vi "main.vi"() -> ()   [LabVIEW 2013]
uses:
  measurement/measurement sweep parameter.ctl
  devices/magnet/magnet polar field.ctl
  devices/magnet/AMI reading polar field.ctl
  app/app global state actions.ctl
  <vilib>/Utility/error.llb/DialogType.ctl
  config.vi
panel:
  in  "Ramp to zero and switch off \nswitch heaters after measurement?":bool=TRUE
  out "Actual T (K)":dbl format="%#_4g"
  out "Current Magnetic\nField\n(430 TCP reading)":T1 {"phi (deg)" format="%#_4g"; "magnitude (T)" format="%#_4g"}
  in  "error in (no error)":errorcluster
  out "Log":string
  out "Current Magnetic Field\n(Gaussmeter reading)":T2 {"theta" format="%#_3g"; "phi" format="%#_3g"; "magnitude" format="%#_3g"}
  out "VNA Sweeping":bool
  out "Magnet Ramping":bool
  out "Sweep Increment":string
  out "Sweep Range":string
  out "Sweep Parameter":T3
  out "Current sweep":string
  in  "Measurement Folder (no backslash at the end)":path=path "D:/UserData/istasinopoulos/VTI/Cu2OSeO3/VTG_1_11_2_14072016/measurement2"
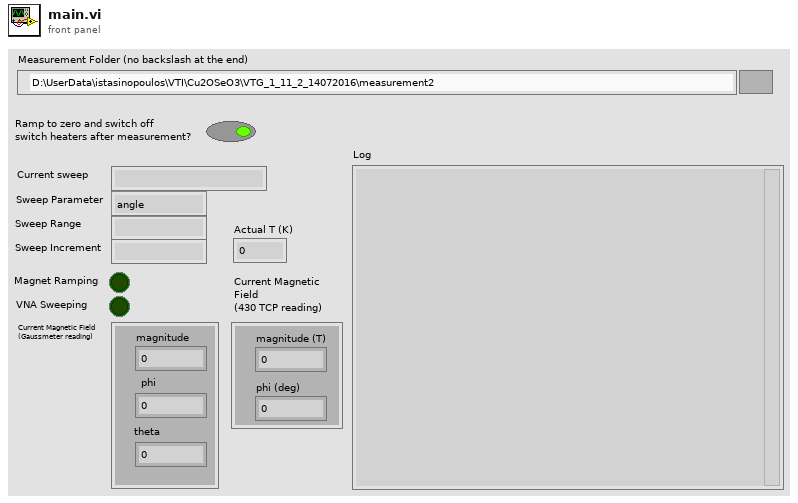
[diagram p1: front panel]
types:
  T1 = typedef "AMI reading polar field.ctl" = cluster{"magnitude (T)":dbl, "phi (deg)":dbl}
  T2 = typedef "magnet polar field.ctl" = cluster{"magnitude":dbl, "phi":dbl, "theta":dbl}
  T3 = typedef "measurement sweep parameter.ctl" = enum16{"angle", "magnetic field"}
  T4 = cluster{"freq start (Hz)":dbl, "freq stop (Hz)":dbl, "power (dBm)":i32, "IF bandwidth (Hz)":dbl, "no. points":i32, "calibration name":string, "SX1":bool, "SX2":bool}
  T5 = typedef "app global state actions.ctl" = enum16{"set field reached", "get cluster", "set cluster", "set current sweep", "set field value", "set 430 TCP reading", "set ramping", "set sweeping", "append log", "clear log", "set finished"}
  T6 = typedef "app global state control.ctl" = cluster{"current field value":T2, "field ramping":bool, "vna sweeping":bool, "Log Messages":string, "current sweep":T7, "measurement finished":bool, "Current Magnetic Field\n(430 TCP reading)":cluster{"magnitude (T)":dbl, "phi (deg)":dbl}, "field was reached":bool}
  T7 = typedef "measconfig cluster.ctl" = cluster{"sweep parameter":T3, "sweep start":dbl, "sweep stop":dbl, "sweep increment":dbl, "temperature":dbl, "path":path, "magnet initial":T2, "magnet reference":T2, "const phi?":bool, "delta phi (deg)":dbl, "delta H (mT)":dbl, "const phi init field?":bool}
  T8 = typedef "DialogType.ctl" = u16
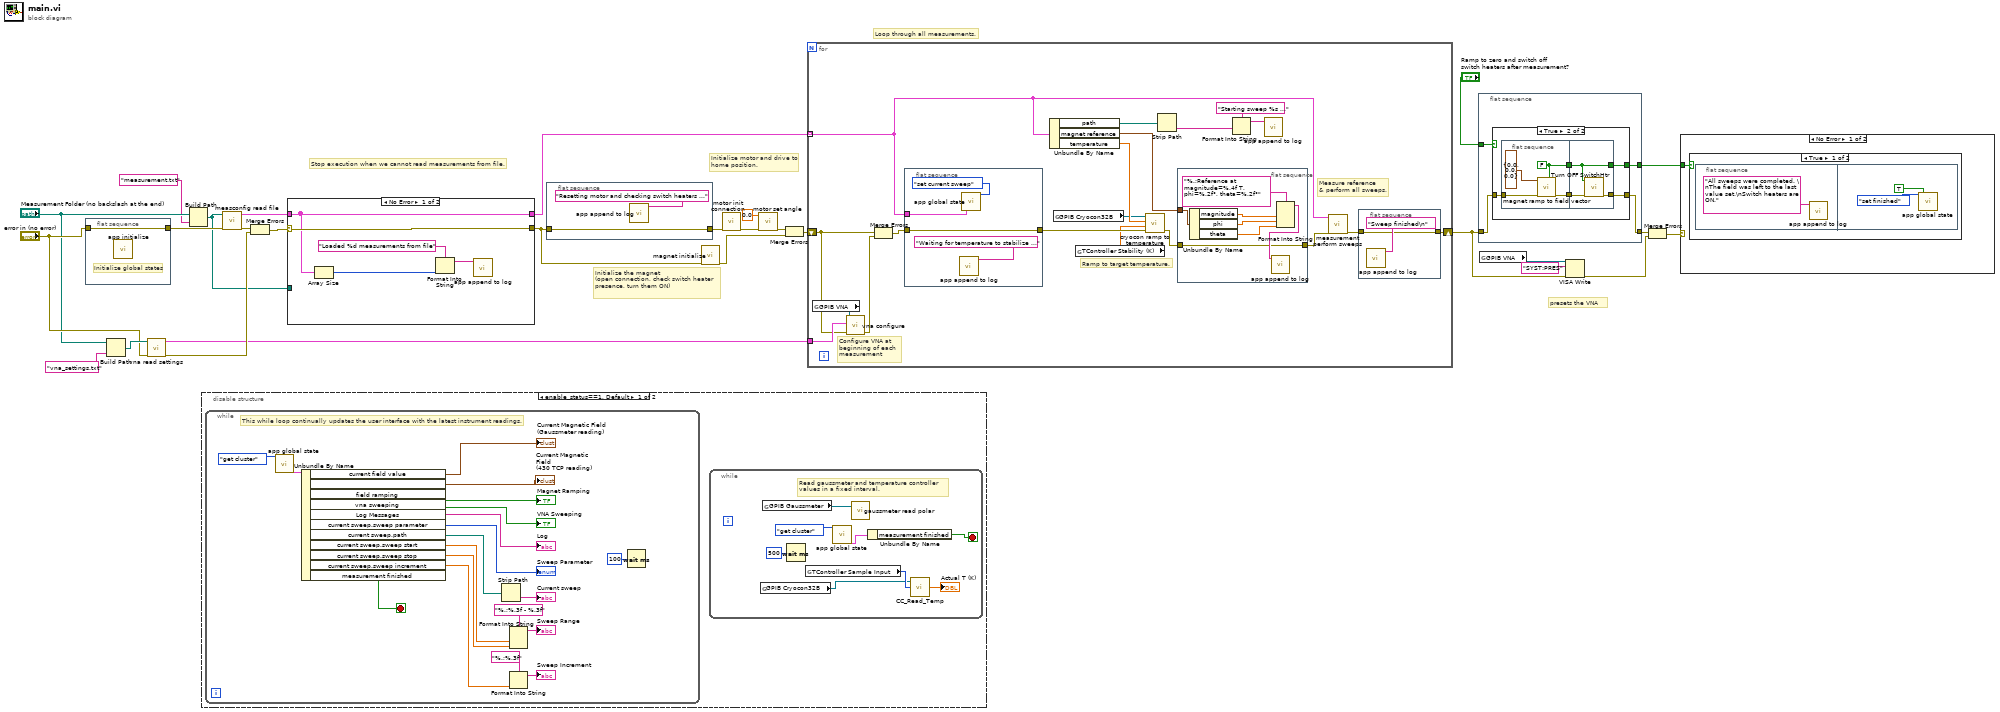
[diagram p0: block diagram]
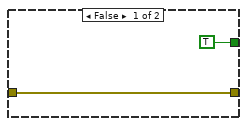
[diagram p2: hidden frame]
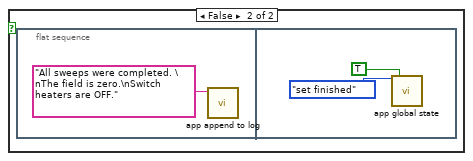
[diagram p4: hidden frame]
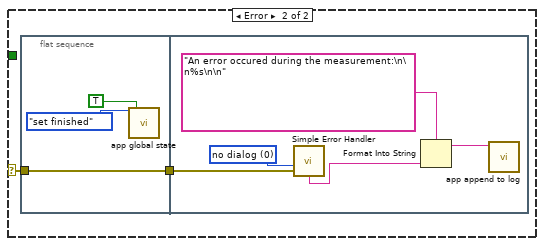
[diagram p5: hidden frame]
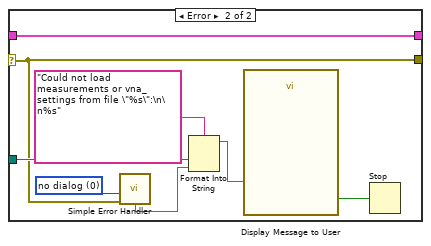
[diagram p6: hidden frame]
diagram:
  # "presets the VNA"
  # "Initialize the magnet \n(open connection, check switch heater presence, turn them ON)"
  # "Loop through all measurements."
  # "Initialize motor and drive to\nhome position."
  # "Stop execution when we cannot read measurements from file."
  n1 = flat-sequence {
    tunnel: "error in (no error)" -> [w29]
    tunnel: [w29] -> w28
    frame #0 {
      # "Initialize global states"
      n2 = call "app initialize.vi"() -> ()  [unwired: 12 in]
    }
  }
  n3 = Build Path(base path="Measurement Folder (no backslash at the end)", name or relative path="vna_settings.txt") -> (appended path=w22:path)
  n4 = call "vna read settings.vi"("error in (no error)"="error in (no error)", "vna settings file"=w22) -> ("error out"=w18:errorcluster, "vna settings"=w1:T4)  [unwired: 8 in]
  n5 = Build Path(base path="Measurement Folder (no backslash at the end)", name or relative path="measurement.txt") -> (appended path=w13:path)
  n6 = disable-structure shown="enable_status==1, Default" {
    frame condition #0 (active) {
      n7 = while {
        stop <- w31 stop-if-true
        # "This while loop continually updates the user interface with the latest instrument readings."
        n8 = call "app global state.vi"("action"=app_global_state_actions."get cluster" ("app global state actions")) -> ("global state"=w47:T6)  [unwired: 18 in]
        n9 = Unbundle By Name(w47) -> ("current field value"=→"Current Magnetic Field\n(Gaussmeter reading)":T2, "Current Magnetic Field\n(430 TCP reading)"=→"Current Magnetic\nField\n(430 TCP reading)":cluster{"magnitude (T)":dbl, "phi (deg)":dbl}, "field ramping"=→"Magnet Ramping":bool, "vna sweeping"=→"VNA Sweeping":bool, "Log Messages"=→"Log":string, "current sweep.sweep parameter"=→"Sweep Parameter":T3, "current sweep.path"=w40:path, "current sweep.sweep start"=w36:dbl, "current sweep.sweep stop"=w35:dbl, "current sweep.sweep increment"=w33:dbl, "measurement finished"=w31:bool)
        n10 = Strip Path(path=w40) -> (name=→"Current sweep":string)  [unwired: 1 out]
        n11 = Format Into String(format string="%.;%.3f - %.3f", w36, w35) -> (resulting string=→"Sweep Range":string)  [unwired: 2 in, 1 out]
        n12 = Format Into String(format string="%.;%.3f", w33) -> (resulting string=→"Sweep Increment":string)  [unwired: 2 in, 1 out]
        n13 = Wait (ms)(milliseconds to wait=u32 100) -> ()  [unwired: 1 out]
      }
      n14 = while {
        stop <- w52 stop-if-true
        # "Read gaussmeter and temperature controller values in a fixed interval."
        n15 = global read "config.vi" "GPIB Cryocon32B"() -> (w50:refnum<visa-resource-name>)
        n16 = global read "config.vi" "GPIB Gaussmeter"() -> (w55:refnum<visa-resource-name>)
        n17 = Wait (ms)(milliseconds to wait=u32 500) -> ()  [unwired: 1 out]
        n18 = global read "config.vi" "TController Sample Input"() -> (w51:u8)
        n19 = call "app global state.vi"("action"=app_global_state_actions."get cluster" ("app global state actions")) -> ("global state"=w54:T6)  [unwired: 18 in]
        n20 = call "gaussmeter read polar.vi"("VISA resource name"=w55) -> ()  [unwired: 8 in, 3 out]
        n21 = Unbundle By Name(w54) -> ("measurement finished"=w52:bool)
        n22 = call <userlib>:"CC_Read_Temp.vi"("Input"=w51, "VISA In"=w50) -> ("Temperature"=→"Actual T (K)":dbl)  [unwired: 1 in, 2 out]
      }
    }
    frame condition #1 {
    }
  }
  n23 = call "measconfig read file.vi"("error in (no error)"=w28, "measurement file"=w13) -> ("error out"=w20:errorcluster, "measurements"=w27:T7[])  [unwired: 8 in]
  n24 = Merge Errors(w20, w18) -> (w19:errorcluster)
  n25 = case shown="No Error" w19 {
    selector: w19 -> [w61 w64]
    tunnel: w27 -> [w59 w69]
    tunnel: [w59 w69] -> w25
    tunnel: [w61 w64] -> w2
    tunnel: w13 -> [_ w67]
    frame No Error {
      n26 = Array Size(array=w59) -> (size(s)=w58:i32)
      n27 = Format Into String(format string="Loaded %d measurements from file", w58) -> (resulting string=w57:string)  [unwired: 2 in, 1 out]
      n28 = call "app append to log.vi"("log line to append"=w57) -> ()  [unwired: 11 in]
    }
    frame Error {
      w63 = T8 0 items=["no dialog", "OK message", "continue or stop message", "OK message + warnings", "continue/stop + warnings"] ("type of dialog (OK msg:1)")
      n29 = call <vilib>:"Simple Error Handler.vi"("type of dialog (OK msg:1)"=w63, "error in (no error)"=w64) -> ("message"=w62:string)  [unwired: 3 in, 4 out]
      n30 = Format Into String(format string="Could not load measurements or vna_settings from file \"%s\":\n\n%s", w67, w62) -> (resulting string=w66:string)  [unwired: 2 in, 1 out]
      n31 = call "Display Message to User"("Message"=w66) -> ("OK"=w65:bool)  [unwired: 9 in, 1 out]
      n32 = Stop(stop? (T)=w65) -> ()
    }
  }
  n33 = flat-sequence {
    tunnel: w2 -> [w71]
    tunnel: [w71] -> w12
    frame #0 {
      n34 = call "app append to log.vi"("log line to append"="Resetting motor and checking switch heaters ...") -> ()  [unwired: 11 in]
    }
  }
  n35 = call "magnet initialize.vi"("error in (no error)"=w2) -> ("error out"=w5:errorcluster)  [unwired: 10 in]
  n36 = call "motor init connection.vi"("error in (no error)"=w12) -> ("error out"=w26:errorcluster)  [unwired: 9 in, 1 out]
  n37 = call "motor set angle.vi"("error in (no error)"=w26, "angle"=0.0) -> ("error out"=w17:errorcluster)  [unwired: 9 in]
  n38 = Merge Errors(w17, w5) -> (w16:errorcluster)
  n39 = for {
    tunnel: w25 -> [w82] mode=indexing
    shift-right: [w85] -> w9
    shift-left: w16 -> [w72]
    tunnel: w1 -> [w74]
    # "Configure VNA at beginning of each measurement"
    # "Measure reference\n& perform all sweeps."
    # "Ramp to target temperature."
    n40 = global read "config.vi" "GPIB VNA"() -> (w75:refnum<visa-resource-name>)
    n41 = call "vna configure.vi"("error in (no error)"=w72, "vna settings"=w74, "VISA resource name"=w75) -> ("error out"=w73:errorcluster)  [unwired: 7 in, 1 out]
    n42 = Merge Errors(w72, w73) -> (w76:errorcluster)
    n43 = flat-sequence {
      tunnel: w76 -> [w101]
      tunnel: [w101] -> w83
      tunnel: w82 -> [w98]
      frame #0 {
        n44 = call "app append to log.vi"("log line to append"="Waiting for temperature to stabilize ...") -> ()  [unwired: 11 in]
        n45 = call "app global state.vi"("action"=app_global_state_actions."set current sweep" ("app global state actions"), "current sweep"=w98) -> ()  [unwired: 17 in, 1 out]
      }
    }
    n46 = Unbundle By Name(w82) -> ("path"=w89:path, "magnet reference"=w79:T2, "temperature"=w90:dbl)
    n47 = global read "config.vi" "GPIB Cryocon32B"() -> (w84:refnum<visa-resource-name>)
    n48 = global read "config.vi" "TController Stability (K)"() -> (w81:dbl)
    n49 = call "cryocon ramp to temperature.vi"("error in (no error)"=w83, "stability (K)"=w81, "target temperature (K)"=w90, "VISA resource name"=w84) -> ("error out"=w80:errorcluster)  [unwired: 6 in, 1 out]
    n50 = Strip Path(path=w89) -> (name=w86:string)  [unwired: 1 out]
    n51 = flat-sequence {
      tunnel: w79 -> [w96]
      tunnel: [w91] -> w77
      tunnel: w80 -> [w91]
      frame #0 {
        n52 = Unbundle By Name(w96) -> ("magnitude"=w95:dbl, "phi"=w94:dbl, "theta"=w93:dbl)
        n53 = Format Into String(format string="%.;Reference at magnitude=%.4f T, phi=%.2f°, theta=%.2f°" ("log line to append"), w95, w94, w93) -> (resulting string=w92:string)  [unwired: 2 in, 1 out]
        n54 = call "app append to log.vi"("log line to append"=w92) -> ()  [unwired: 11 in]
      }
    }
    n55 = Format Into String(format string="Starting sweep %s ...", w86) -> (resulting string=w87:string)  [unwired: 2 in, 1 out]
    n56 = call "app append to log.vi"("log line to append"=w87) -> ()  [unwired: 11 in]
    n57 = call "measurement perform sweeps.vi"("error in (no error)"=w77, "measurement definition"=w82) -> ("error out"=w78:errorcluster)  [unwired: 9 in]
    n58 = flat-sequence {
      tunnel: w78 -> [w102]
      tunnel: [w102] -> w85
      frame #0 {
        n59 = call "app append to log.vi"("log line to append"="Sweep finished\n") -> ()  [unwired: 11 in]
      }
    }
  }
  n60 = flat-sequence {
    tunnel: w9 -> [w106]
    tunnel: [w105] -> w11
    tunnel: "Ramp to zero and switch off \nswitch heaters after measurement?" -> [w107]
    tunnel: [w104] -> w3
    frame #0 {
      n61 = case shown="True" w107 {
        tunnel: w106 -> [w109 w114]
        tunnel: [w109 w110] -> w105
        tunnel: [TRUE ("measurement finished") w113] -> w104
        frame False {
        }
        frame True {
          n62 = flat-sequence {
            tunnel: w114 -> [w117]
            tunnel: [w115] -> w112
            tunnel: [w118] -> w111
            tunnel: [w120] -> w110
            tunnel: [w119] -> w113
            tunnel: w112 -> [w119]
            tunnel: w111 -> [w121]
            frame #0 {
              w115 = FALSE ("measurement finished")
              n63 = call "magnet ramp to field vector.vi"("const phi?"=w115, "error in (no error)"=w117, "magnet polar"=T2 {"magnitude"=0.0, "phi"=0.0, "theta"=0.0} ("magnet initial")) -> ("error out"=w118:errorcluster)  [unwired: 6 in, 1 out]
            }
            frame #1 {
              n64 = call "Turn OFF SwitchHtr.vi"("error in (no error)"=w121, "Turn ON / OFF"=w119) -> ("error out"=w120:errorcluster)  [unwired: 7 in, 2 out]
            }
          }
        }
      }
    }
  }
  n65 = global read "config.vi" "GPIB VNA"() -> (w7:refnum<visa-resource-name>)
  n66 = VISA Write(VISA resource name=w7, write buffer="SYST:PRES", error in (no error)=w9) -> (error out=w8:errorcluster)  [unwired: 2 out]
  n67 = Merge Errors(w11, w8) -> (w10:errorcluster)
  n68 = case shown="No Error" w10 {
    selector: w10 -> [_ w130]
    tunnel: w3 -> [w122 _]
    frame No Error {
      n69 = case shown="True" w122 {
        frame True {
          n70 = flat-sequence {
            frame #0 {
              n71 = call "app append to log.vi"("log line to append"="All sweeps were completed. \nThe field was left to the last value set.\nSwitch heaters are ON.") -> ()  [unwired: 11 in]
            }
            frame #1 {
              n72 = call "app global state.vi"("action"=app_global_state_actions."set finished" ("app global state actions"), "measurement finished"=TRUE) -> ()  [unwired: 17 in, 1 out]
            }
          }
        }
        frame False {
          n73 = flat-sequence {
            frame #0 {
              n74 = call "app append to log.vi"("log line to append"="All sweeps were completed. \nThe field is zero.\nSwitch heaters are OFF.") -> ()  [unwired: 11 in]
            }
            frame #1 {
              n75 = call "app global state.vi"("action"=app_global_state_actions."set finished" ("app global state actions"), "measurement finished"=TRUE) -> ()  [unwired: 17 in, 1 out]
            }
          }
        }
      }
    }
    frame Error {
      n76 = flat-sequence {
        tunnel: w130 -> [w133]
        tunnel: [w133] -> w129
        tunnel: w129 -> [w134]
        frame #0 {
          n77 = call "app global state.vi"("action"=app_global_state_actions."set finished" ("app global state actions"), "measurement finished"=TRUE) -> ()  [unwired: 17 in, 1 out]
        }
        frame #1 {
          w138 = T8 0 items=["no dialog", "OK message", "continue or stop message", "OK message + warnings", "continue/stop + warnings"] ("type of dialog (OK msg:1)")
          n78 = call <vilib>:"Simple Error Handler.vi"("type of dialog (OK msg:1)"=w138, "error in (no error)"=w134) -> ("message"=w135:string)  [unwired: 3 in, 4 out]
          n79 = Format Into String(format string="An error occured during the measurement:\n\n%s\n\n", w135) -> (resulting string=w136:string)  [unwired: 2 in, 1 out]
          n80 = call "app append to log.vi"("log line to append"=w136) -> ()  [unwired: 11 in]
        }
      }
    }
  }
